vi "SVT Human Vibration Weighting Filter (frequency) (1 Ch).vi"(0 "spectrum":cluster{"f0":dbl, "df":dbl, "magnitude":dbl[]} {"magnitude" format="%.2p"; "df" format="%.2p"; "f0" format="%.2p"}, 1 "weighting":u16(ring) items=["Linear"=0, "Wh: hand-arm"=13, "Wb: vertical whole-body"=8, "Wc: horizontal whole-body"=9, "Wd: horizontal whole-body"=10, "We: rotational whole-body"=11, "Wj: vertical head"=14, "Wk: vertical whole-body"=15, "Wm: whole-body in buildings"=16, "Wf: low-frequency whole-body"=12], 4 "spectrum info in":T1={"channel name"="", "description"="", "x-axis units"=0, "spectral info"={"spectrum type"=enum."Power [Magnitude^2]", "linear/dB"=enum."linear", "window"=0, "window size"=0, "FFT size"=0}, "engineering units"=0, "custom label"="", "dB reference [EU]"=0.0, "peak units"=enum."rms", "weighting filter"=0, "spectral density?"=FALSE, "unit label"="", "spectrum skewed?"=FALSE, "complimentary spectrum units"=enum."none"} {"x-axis units" items=["Time (s)"=0, "Frequency-CB (Hz)"=1, "Frequency-CPB (Hz)"=1248, "Frequency-Arbitrary (Hz)"=2357, "Quefrency (s)"=2, "Revolutions (rev)"=3, "Order"=4, "Speed (RPM)"=11, "Speed (rad/s)"=21, "Index"=65535]; "weighting filter" items=["Linear", "A-weighting", "B-weighting", "C-weighting", "ITU-R 468-4", "Dolby", "CCITT", "C-message", "Wb", "Wc", "Wd", "We", "Wf", "Wh", "Wj", "Wk", "Wm", "AES17 20 kHz lowpass", "AES17 40 kHz lowpass", "AES17 20 kHz highpass", "AES17 40 kHz highpass"]; "dB reference [EU]" format="%.2f"; "engineering units" items=["custom..."=0, "V"=1, "A"=21, "C"=30, "pC"=31, "s"=32, "-"=29, "Pa"=2, "N"=20, "g"=3, "m/s^2"=4, "m/s"=5, "m"=6, "mm/s"=12, "mm"=13, "micron/s"=14, "micron"=15, "in/s^2"=7, "in/s"=8, "in"=9, "mil/s"=10, "mil"=11, "rad/s^2"=16, "rad/s"=17, "rad"=18, "deg/s^2"=26, "deg/s"=27, "deg"=28, "RPM"=22, "cycle/s^2"=23, "Hz"=24, "cycle"=25, "strain"=19]; "spectral info"."window" items=["None "=0, "Hanning"=1, "Hamming"=2, "Blackman-Harris"=3, "Exact Blackman"=4, "Blackman"=5, "Flat Top"=6, "4 Term B-Harris "=7, "7 Term B-Harris"=8, "Low Sidelobe"=9, "Force - Exponential"=10, "Gaussian"=62]}, 5 "error in (no error)":errorcluster) -> (14 "weighted spectrum":cluster{"f0":dbl, "df":dbl, "magnitude":dbl[]} {"magnitude" format="%.2p"; "df" format="%.2p"; "f0" format="%.2p"}, 15 "unit label":string, 18 "spectrum info out":T1={"channel name"="", "description"="", "x-axis units"=0, "spectral info"={"spectrum type"=enum."Power [Magnitude^2]", "linear/dB"=enum."linear", "window"=0, "window size"=0, "FFT size"=0}, "engineering units"=0, "custom label"="", "dB reference [EU]"=0.0, "peak units"=enum."rms", "weighting filter"=0, "spectral density?"=FALSE, "unit label"="", "spectrum skewed?"=FALSE, "complimentary spectrum units"=enum."none"} {"x-axis units" items=["Time (s)"=0, "Frequency-CB (Hz)"=1, "Frequency-CPB (Hz)"=1248, "Frequency-Arbitrary (Hz)"=2357, "Quefrency (s)"=2, "Revolutions (rev)"=3, "Order"=4, "Speed (RPM)"=11, "Speed (rad/s)"=21, "Index"=65535]; "weighting filter" items=["Linear", "A-weighting", "B-weighting", "C-weighting", "ITU-R 468-4", "Dolby", "CCITT", "C-message", "Wb", "Wc", "Wd", "We", "Wf", "Wh", "Wj", "Wk", "Wm", "AES17 20 kHz lowpass", "AES17 40 kHz lowpass", "AES17 20 kHz highpass", "AES17 40 kHz highpass"]; "dB reference [EU]" format="%.2f"; "engineering units" items=["custom..."=0, "V"=1, "A"=21, "C"=30, "pC"=31, "s"=32, "-"=29, "Pa"=2, "N"=20, "g"=3, "m/s^2"=4, "m/s"=5, "m"=6, "mm/s"=12, "mm"=13, "micron/s"=14, "micron"=15, "in/s^2"=7, "in/s"=8, "in"=9, "mil/s"=10, "mil"=11, "rad/s^2"=16, "rad/s"=17, "rad"=18, "deg/s^2"=26, "deg/s"=27, "deg"=28, "RPM"=22, "cycle/s^2"=23, "Hz"=24, "cycle"=25, "strain"=19]; "spectral info"."window" items=["None "=0, "Hanning"=1, "Hamming"=2, "Blackman-Harris"=3, "Exact Blackman"=4, "Blackman"=5, "Flat Top"=6, "4 Term B-Harris "=7, "7 Term B-Harris"=8, "Low Sidelobe"=9, "Force - Exponential"=10, "Gaussian"=62]}, 19 "error out":errorcluster)   [LabVIEW 2017, in "SoundVib_HumanVibration.lvlib"]
doc: "Applies the selected human vibration weighting to FFT-based spectra. This VI weights each spectral bin according to the attenuation of the specified filter at the bin center frequency. This VI does not maintain state internally; you can use this VI in a loop to process multiple blocks. Wire data to the <B>spectrum</B> input to determine the polymorphic instance to use or manually select the instance."
uses:
  <vilib>/addons/Sound and Vibration/svt_Weighting/SoundVib_HumanVibration.lvlib
  <vilib>/addons/_NISVFA/_Shared subVIs/Controls/svc_Spectrum Info.ctl
  <vilib>/addons/_NISVFA/_Shared subVIs/Controls/svc_X-Axis Units.ctl
  <vilib>/addons/_NISVFA/_Shared subVIs/Controls/svc_Spectrum Type.ctl
  <vilib>/addons/_NISVFA/_Shared subVIs/Controls/svc_Engineering Units Text Ring.ctl
  <vilib>/addons/_NISVFA/_Shared subVIs/Controls/svc_Weighting Filter Text Ring.ctl
  <vilib>/addons/_NISVFA/_Shared subVIs/Controls/svc_Complimentary Spectrum Units.ctl
  <vilib>/addons/_NISVFA/_Shared subVIs/Common/svc_Get Weighting Enum and Labels.vi
  <vilib>/addons/_NISVFA/_Shared subVIs/Common/svc_Unit Label Lexical Class.vi
  <vilib>/addons/_NISVFA/_Shared subVIs/Common/svc_Engineering Units to Unit Label.vi
  <vilib>/addons/_NISVFA/_Shared subVIs/Common/svc_Format Value (DBL).vi
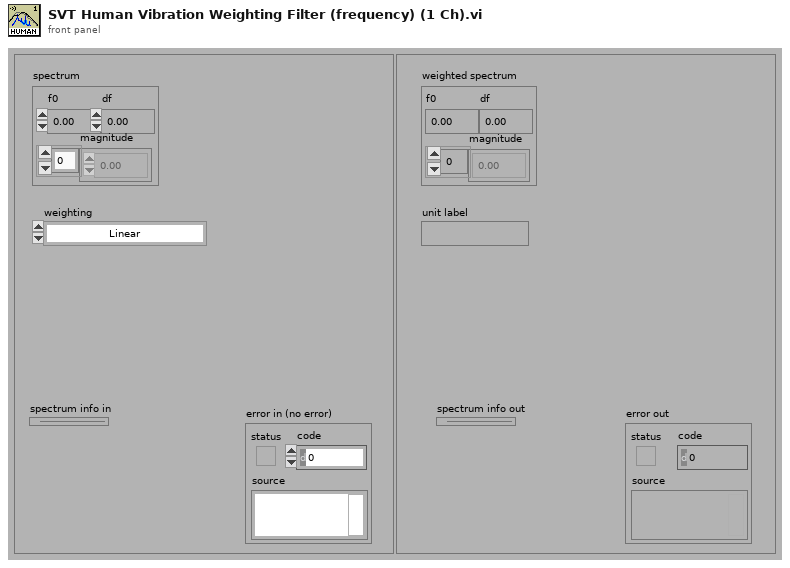
[diagram p1: front panel]
types:
  T1 = typedef "svc_Spectrum Info.ctl" = cluster{"channel name":string, "description":string, "x-axis units":T2, "spectral info":cluster{"spectrum type":T3, "linear/dB":enum16{"linear", "dB"}, "window":u16, "window size":i32, "FFT size":i32}, "engineering units":T4, "custom label":string, "dB reference [EU]":dbl, "peak units":enum16{"rms", "peak", "peak-peak"}, "weighting filter":T5, "spectral density?":bool, "unit label":string, "spectrum skewed?":bool, "complimentary spectrum units":T6}
  T2 = typedef "svc_X-Axis Units.ctl" = u16
  T3 = typedef "svc_Spectrum Type.ctl" = enum16{"FFT Spectrum [complex]", "Amplitude [Magnitude]", "Power [Magnitude^2]", "Cross Spectrum [complex]", "Frequency Response [Complex]"}
  T4 = typedef "svc_Engineering Units Text Ring.ctl" = u16
  T5 = typedef "svc_Weighting Filter Text Ring.ctl" = u16
  T6 = typedef "svc_Complimentary Spectrum Units.ctl" = enum16{"none", "radians", "degrees", "cycles", "imaginary"}
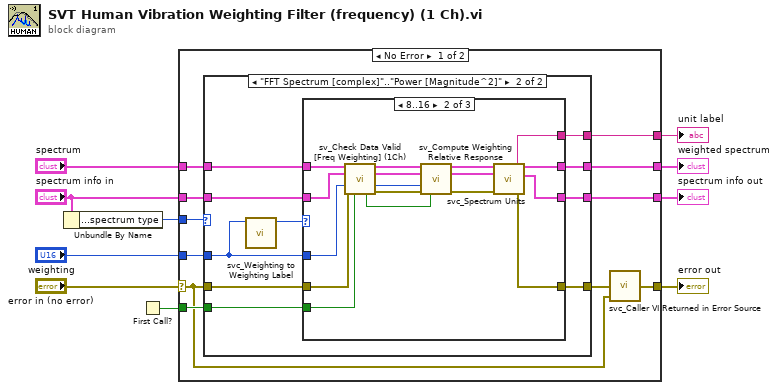
[diagram p0: block diagram]
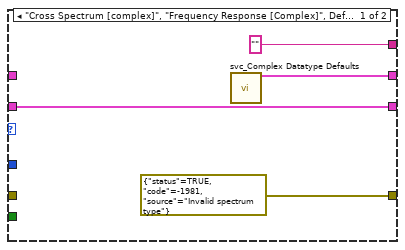
[diagram p2: hidden frame]
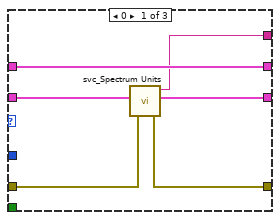
[diagram p3: hidden frame]
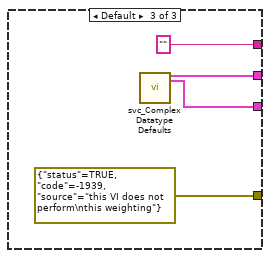
[diagram p4: hidden frame]
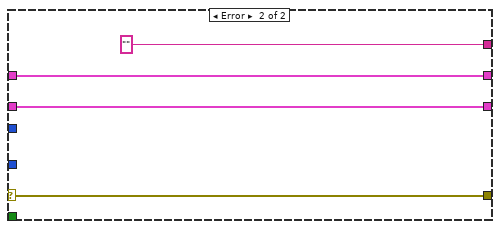
[diagram p5: hidden frame]
diagram:
  n1 = Unbundle By Name("spectrum info in") -> ("spectral info.spectrum type"=w2:T3)
  n2 = First Call?() -> (First Call?: T/F=w1:bool)
  n3 = case shown="No Error" "error in (no error)" {
    selector: "error in (no error)" -> [w11 w65]
    tunnel: [w19 w62] -> w10
    tunnel: "weighting" -> [w21 _]
    tunnel: "spectrum" -> [w20 w62]
    tunnel: [w17 w65] -> w7
    tunnel: [w15 "" ("dB label")] -> w6
    tunnel: "spectrum info in" -> [w18 w63]
    tunnel: [w16 w63] -> w4
    tunnel: w2 -> [w13 _]
    tunnel: w1 -> [w12 _]
    frame No Error {
      n4 = case shown="\"FFT Spectrum [complex]\"..\"Power [Magnitude^2]\"" w13 {
        tunnel: w21 -> [_ w27]
        tunnel: w20 -> [_ w29]
        tunnel: [w22 w35] -> w19
        tunnel: w18 -> [w23 w28]
        tunnel: w11 -> [_ w31]
        tunnel: [w23 w34] -> w16
        tunnel: ["" ("unit label") w33] -> w15
        tunnel: [errorcluster {"status"=TRUE, "code"=-1981, "source"="Invalid spectrum type"} ("error out") w32] -> w14
        tunnel: w12 -> [_ w30]
        frame "Cross Spectrum [complex]", "Frequency Response [Complex]", Default {
          n5 = call <vilib>:"svc_Complex Datatype Defaults.vi"() -> ("empty spectrum"=w22:cluster{"f0":dbl, "df":dbl, "magnitude":dbl[]})  [unwired: 11 in, 8 out]
        }
        frame "FFT Spectrum [complex]".."Power [Magnitude^2]" {
          n6 = call <vilib>:"svc_Weighting to Weighting Label.vi"("weighting filter"=w27) -> ("weighting enum"=w26:T5)  [unwired: 9 in, 1 out]
          n7 = case shown="8..16" w26 {
            tunnel: [w41 w57 w61] -> w35
            tunnel: [w38 w56 w60] -> w34
            tunnel: [w36 w55 "" ("unit label")] -> w33
            tunnel: [w37 w53 errorcluster {"status"=TRUE, "code"=-1939, "source"="this VI does not perform\nthis weighting"} ("error out")] -> w32
            tunnel: w31 -> [w40 w52 _]
            tunnel: w30 -> [_ w50 _]
            tunnel: w29 -> [w41 w49 _]
            tunnel: w27 -> [_ w47 _]
            tunnel: w28 -> [w39 w45 _]
            frame 0 {
              n8 = call <vilib>:"svc_Spectrum Units.vi"("error in (no error)"=w40, "spectrum info in"=w39) -> ("error out"=w37:errorcluster, "spectrum info out"=w38:T1, "unit label"=w36:string)  [unwired: 2 in, 1 out]
            }
            frame 8..16 {
              n9 = call <vilib>:"sv_Check Data Valid [Freq Weighting] (1Ch).vi"("spectrum"=w49, "spectrum info"=w45, "weighting filter"=w47, "error in (no error)"=w52, "reset in"=w50) -> ("dup spectrum"=w48:cluster{"f0":dbl, "df":dbl, "Spectrum":dbl[]}, "dup spectrum info"=w46:T1, "dup weighting filter"=w43:T5, "reset out"=w44:bool, "error out"=w51:errorcluster)  [unwired: 6 in]
              n10 = call <vilib>:"sv_Compute Weighting Relative Response.vi"("spectrum"=w48, "spectrum info"=w46, "weighting filter"=w43, "error in (no error)"=w51, "reset"=w44) -> ("weighted spectrum"=w57:cluster{"f0":dbl, "df":dbl, "Spectrum":dbl[]}, "spectrum info out"=w42:T1, "error out"=w54:errorcluster)  [unwired: 8 in]
              n11 = call <vilib>:"svc_Spectrum Units.vi"("error in (no error)"=w54, "spectrum info in"=w42) -> ("error out"=w53:errorcluster, "spectrum info out"=w56:T1, "unit label"=w55:string)  [unwired: 2 in, 1 out]
            }
            frame Default {
              n12 = call <vilib>:"svc_Complex Datatype Defaults.vi"() -> ("empty spectrum"=w61:cluster{"f0":dbl, "df":dbl, "magnitude":dbl[]}, "dead spectrum info"=w60:T1)  [unwired: 11 in, 7 out]
            }
          }
        }
      }
      n13 = call <vilib>:"svc_Caller VI Returned in Error Source.vi"("warning input to caller"=w11, "error in (no error)"=w14) -> ("error out"=w17:errorcluster)  [unwired: 3 in]
    }
    frame Error {
    }
  }
  "error out" <- w7
  "weighted spectrum" <- w10
  "unit label" <- w6
  "spectrum info out" <- w4
